vi "Ini.vi"(8 "error in":errorcluster, 11 "INI file path":path=path "C:/Users/user/Documents/GitHub/AADXB08/AADXB08_LV/data/AADXB08.ini") -> (0 "DBlink":string, 2 "PLC_IP":string, 3 "Mode":u32)   [LabVIEW 2019]
uses:
  <vilib>/Utility/config.llb/Read Key (U32).vi
  <vilib>/Utility/config.llb/Read Key (String).vi
  <vilib>/Utility/config.llb/NI_LVConfig.lvlib
panel:
  out "error out":errorcluster
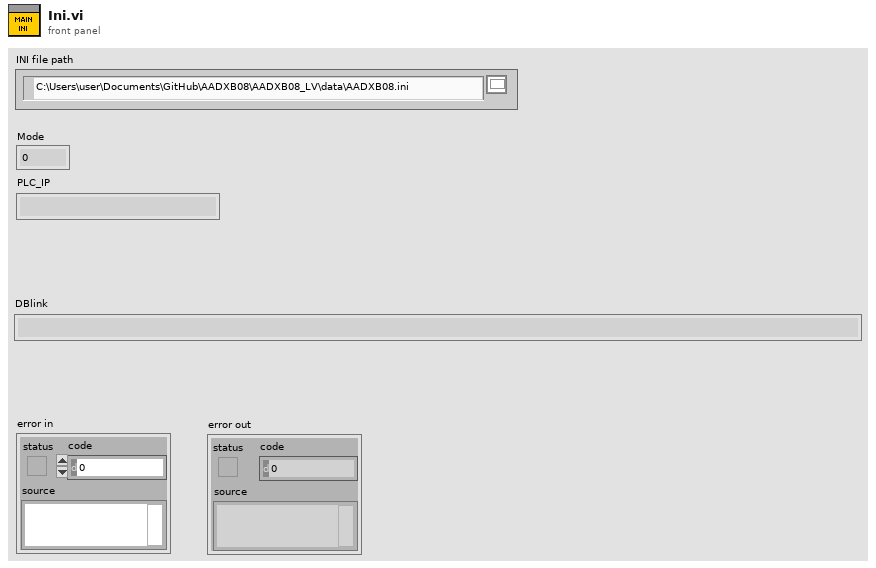
[diagram p1: front panel]
types:
  T1 = typedef "NI_LVConfig.lvlib/Config Data RefNum.ctl" = refnum<k1>
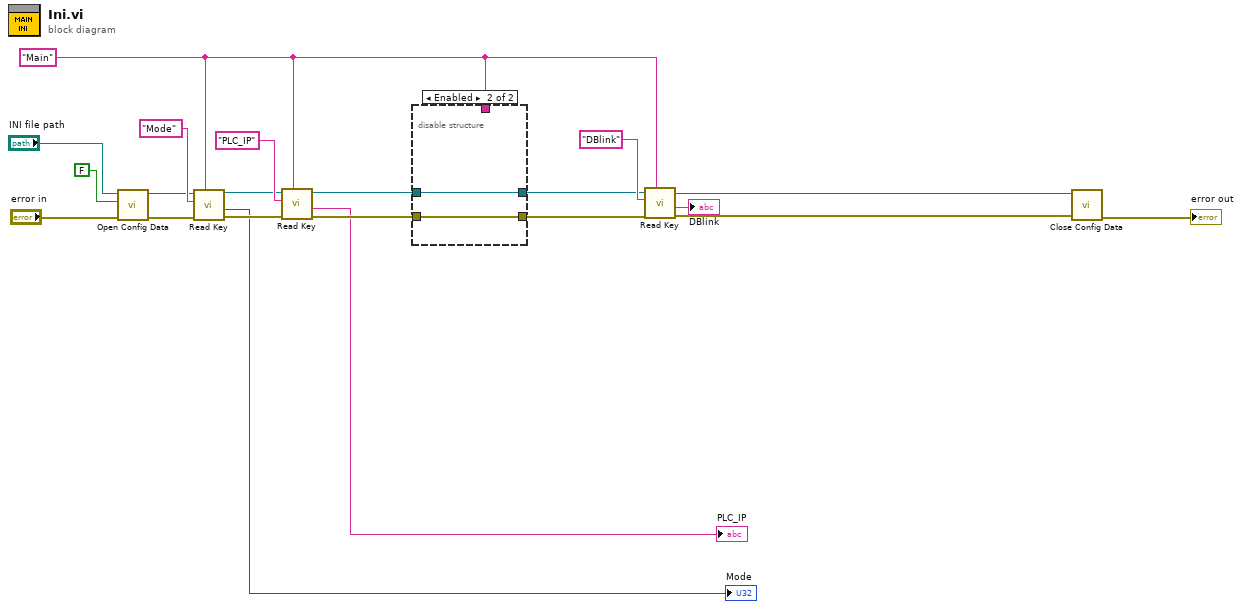
[diagram p0: block diagram]
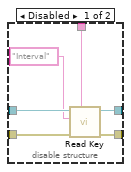
[diagram p2: hidden frame]
diagram:
  w4 = "Main" ("Main section")
  n1 = call <vilib>:"Open Config Data.vi"("error in (no error)"="error in", "create file if necessary (T)"=FALSE ("create file if necessary? (T)"), "configuration file path"="INI file path") -> ("error out"=w19:errorcluster, "refnum"=w17:T1)  [unwired: 6 in, 1 out]
  n2 = call-poly <vilib>:"Read Key.vi"("section"=w4, "error in (no error)"=w19, "key"="Mode", "refnum"=w17) -> ("error out"=w12:errorcluster, "value"=→"Mode":u32, "refnum out"=w13:T1)  [unwired: 1 in, 4 out]
  n3 = call-poly <vilib>:"Read Key.vi"("section"=w4, "error in (no error)"=w12, "key"="PLC_IP", "refnum"=w13) -> ("error out"=w10:errorcluster, "value"=→"PLC_IP":string, "refnum out"=w11:T1)  [unwired: 2 in, 3 out]
  n4 = disable-structure shown="Enabled" {
    disable-tunnel: w11 -> [w27 w29]
    disable-tunnel: w10 -> [w26 w28]
    disable-tunnel: [w24 w29] -> w6
    disable-tunnel: [w23 w28] -> w5
    disable-tunnel: w4 -> [w22 _]
    frame Disabled {
      n5 = call-poly <vilib>:"Read Key.vi"("section"=w22, "error in (no error)"=w26, "key"="Interval", "refnum"=w27) -> ("error out"=w23:errorcluster, "refnum out"=w24:T1)  [unwired: 1 in, 5 out]
    }
    frame Enabled {
    }
  }
  n6 = call-poly <vilib>:"Read Key.vi"("section"=w4, "error in (no error)"=w5, "key"="DBlink", "refnum"=w6) -> ("error out"=w3:errorcluster, "value"=→"DBlink":string, "refnum out"=w2:T1)  [unwired: 2 in, 3 out]
  n7 = call <vilib>:"Close Config Data.vi"("error in (no error)"=w3, "refnum"=w2) -> ("error out"=→"error out":errorcluster)  [unwired: 1 in, 8 out]
